vi "Write NewData Msg.vi"(10 "TouchScreen.lvlib:NewData Msg.lvclass":refnum<class "NewData Msg.lvclass">, 11 "TouchScreen in":refnum<class "TouchScreen.lvclass">) -> (3 "TouchScreen out":refnum<class "TouchScreen.lvclass">)   [LabVIEW 2020, in "TouchScreen.lvlib" / "TouchScreen.lvclass"]
uses:
  TouchScreen.lvclass
  TouchScreen Messages/NewData Msg/NewData Msg.lvclass
  TouchScreen.lvclass/TouchScreen.ctl
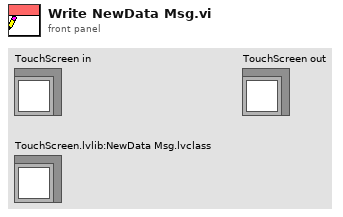
[diagram p1: front panel]
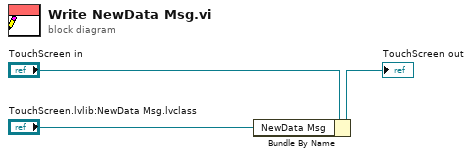
[diagram p0: block diagram]
diagram:
  n1 = Bundle By Name(cluster="TouchScreen in", "NewData Msg"="TouchScreen.lvlib:NewData Msg.lvclass") -> (→"TouchScreen out":refnum<class "TouchScreen.lvclass">)
